vi "Untitled 1.vi"   [LabVIEW 2012]
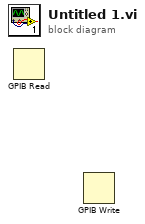
[diagram p0: block diagram]
diagram:
  n1 = GPIB Read() -> ()  [unwired: 5 in, 3 out]
  n2 = GPIB Write() -> ()  [unwired: 5 in, 2 out]
